vi "Read Read Only.vi"(8 "error in (no error)":errorcluster, 11 "Const_Time in":refnum<class "Const_Time.lvclass">) -> (0 "error out":errorcluster, 2 "Read Only":bool, 3 "Const_Time out":refnum<class "Const_Time.lvclass">)   [LabVIEW 2021, in "Const_Time.lvclass"]
uses:
  Const_Time.lvclass
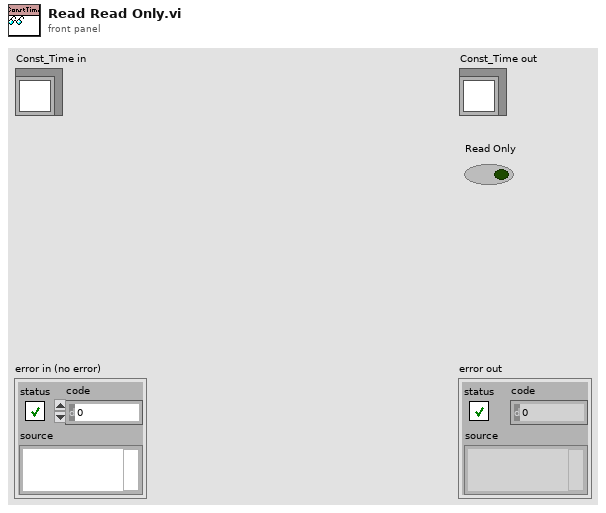
[diagram p1: front panel]
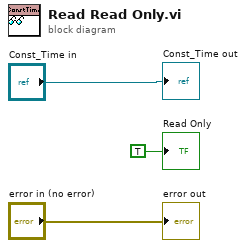
[diagram p0: block diagram]
diagram:
  "error out" <- "error in (no error)"
  "Const_Time out" <- "Const_Time in"
  "Read Only" <- TRUE ("Read Only")
